vi "kf_update.vi"(8 "z":T1, 9 "u":T1, 11 "KF in":T2={"A"=[], "B"=[], "H"=[], "Q"=[], "R"=[], "x"=[], "P"=[], "x lim"=[], "y lim"=[], "K"=[], "Converge count"=-1} {"K" format="%#_3g"; "y lim" format="%#_3g"; "x lim" format="%#_3g"; "P" format="%#_3g"; "H" format="%#_3g"; "x" format="%#_3g"; "Q" format="%#_3g"; "R" format="%#_3g"; "B" format="%#_3g"; "A" format="%#_3g"}) -> (0 "y":T1, 3 "KF out":T2={"A"=[], "B"=[], "H"=[], "Q"=[], "R"=[], "x"=[], "P"=[], "x lim"=[], "y lim"=[], "K"=[], "Converge count"=-1} {"K" format="%#_3g"; "y lim" format="%#_3g"; "x lim" format="%#_3g"; "P" format="%#_3g"; "H" format="%#_3g"; "x" format="%#_3g"; "Q" format="%#_3g"; "R" format="%#_3g"; "B" format="%#_3g"; "A" format="%#_3g"})   [LabVIEW 2014]
uses:
  <vilib>/Analysis/Matrix/Datatypes/RealMatrix.ctl
  kalman_filter.ctl
  <vilib>/Analysis/baseanly.llb/Real A x B.vi
  <vilib>/Analysis/Matrix/Numeric/Add/Add - RM,RM.vi
  <vilib>/Analysis/Matrix/Numeric/Subtract/Subtract - RM,RM.vi
  <vilib>/Analysis/NI_AALBase.lvlib
  <vilib>/Analysis/Matrix/NI_Matrix.lvlib
panel:
  # "Command input.  If empty, this is the same as an appropriate dimension matrix of zeros."
  # "Measurement residue"
  # "Measurement."
  # "Something not exactly standard here is that the state (x) is a 2D array.  In the case where there is only one column, then this degenerates to the standard KF.  If there are multiple columns, then each column is an independent filter with identical structure and parameters (sometimes called block update).  When there are many independent axes this is significantly more efficient than the standard approach of concatenating independent systems on the diagonal.  It's also clearer because the parameter matrices end up much smaller, with fewer zero entries and less duplicated structure.\n\nBecause of this, the command input (u) and the measurement (z) are also 2D, with each column being the command or measurements for the corresponding filter."
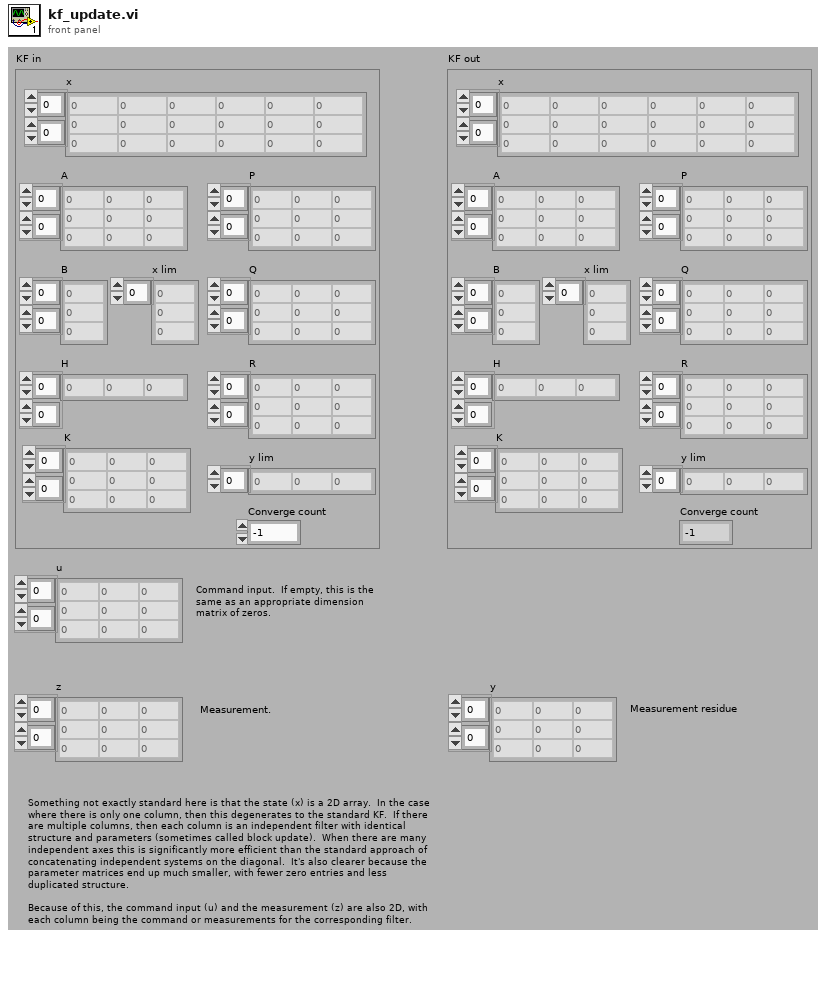
[diagram p1: front panel]
types:
  T1 = typedef "NI_Matrix.lvlib/RealMatrix.ctl" = dbl[][]
  T2 = typedef "kalman_filter.ctl" = cluster{"A":T1, "B":T1, "H":T1, "Q":T1, "R":T1, "x":T1, "P":T1, "x lim":dbl[], "y lim":dbl[], "K":T1, "Converge count":i32}
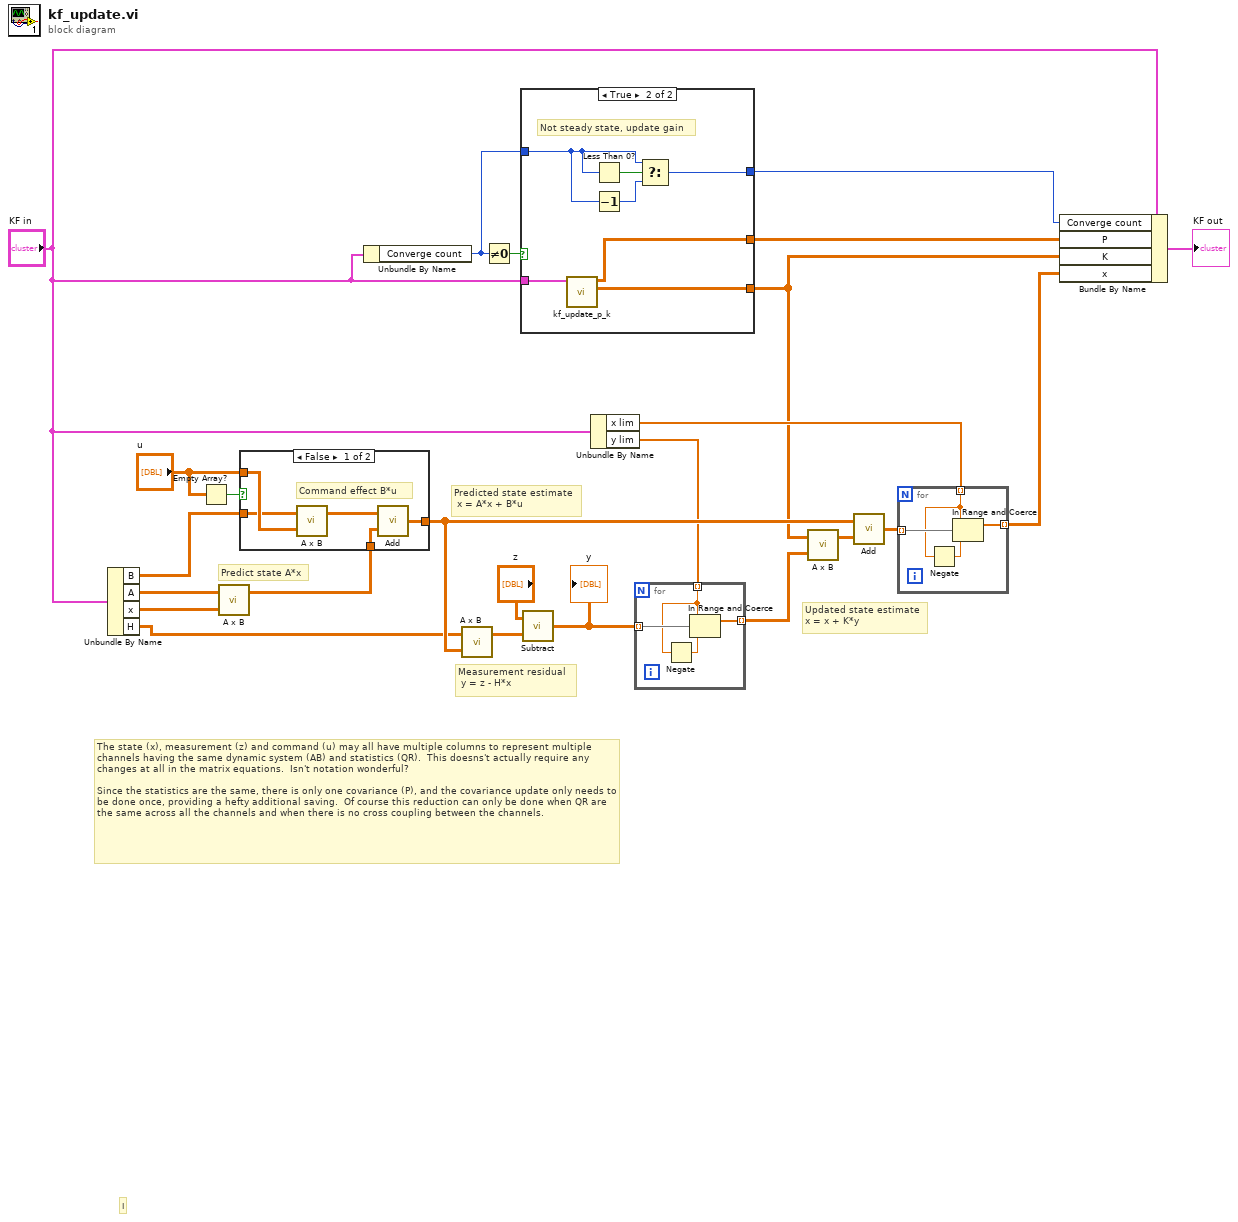
[diagram p0: block diagram]
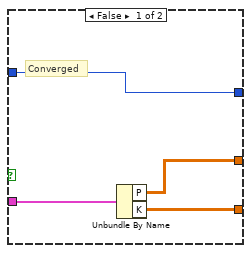
[diagram p2: hidden frame]
diagram:
  # "The state (x), measurement (z) and command (u) may all have multiple columns to represent multiple channels having the same dynamic system (AB) and statistics (QR).  This doesns't actually require any changes at all in the matrix equations.  Isn't notation wonderful?  \n\nSince the statistics are the same, there is only one covariance (P), and the covariance update only needs to be done once, providing a hefty additional saving.  Of course this reduction can only be done when QR are the same across all the channels and when there is no cross coupling between the channels."
  # "Updated state estimate\nx = x + K*y"
  # "Measurement residual\n y = z - H*x"
  # "Predicted state estimate\n x = A*x + B*u"
  # "Predict state A*x"
  # "I"
  n1 = Unbundle By Name("KF in") -> ("B"=w15:T1, "A"=w16:T1, "x"=w17:T1, "H"=w14:T1)
  n2 = Empty Array?(array="u") -> (empty?=w7:bool)
  n3 = call-poly <vilib>:"A x B.vi"("B"=w17, "A"=w16) -> ("A x B"=w20:T1)  [unwired: 1 out]
  n4 = case shown="False" w7 {
    tunnel: [w28 w30] -> w22
    tunnel: "u" -> [w27 _]
    tunnel: w20 -> [w26 w30]
    tunnel: w15 -> [w25 _]
    frame False {
      # "Command effect B*u"
      n5 = call-poly <vilib>:"A x B.vi"("B"=w27, "A"=w25) -> ("A x B"=w29:T1)  [unwired: 1 out]
      n6 = call-poly <vilib>:"Add.vi"("Real Matrix B"=w26, "Real Matrix A"=w29) -> ("A + B"=w28:T1)
    }
    frame True {
    }
  }
  n7 = Unbundle By Name("KF in") -> ("Converge count"=w3:i32)
  n8 = call-poly <vilib>:"A x B.vi"("B"=w22, "A"=w14) -> ("A x B"=w23:T1)  [unwired: 1 out]
  n9 = Not Equal To 0?(x=w3) -> (x != 0?=w4:bool)
  n10 = case shown="True" w4 {
    tunnel: [w33 w41] -> w1
    tunnel: [w32 w40] -> w19
    tunnel: "KF in" -> [w31 w39]
    tunnel: w3 -> [w34 w36]
    tunnel: [w34 w35] -> w2
    frame False {
      # "Converged"
      n11 = Unbundle By Name(w31) -> ("P"=w32:T1, "K"=w33:T1)
    }
    frame True {
      # "Not steady state, update gain"
      n12 = call "kf_update_p_k.vi"("KF in"=w39) -> ("K"=w41:T1, "P"=w40:T1)  [unwired: 9 in]
      n13 = Less Than 0?(x=w36) -> (x < 0?=w38:bool)
      n14 = Decrement(x=w36) -> (x-1=w37:i32)
      n15 = Select(t=w36, s=w38, f=w37) -> (s? t:f=w35:i32)
    }
  }
  n16 = call-poly <vilib>:"Subtract.vi"("Real Matrix B"=w23, "Real Matrix A"="z") -> ("A - B"=w11:T1)
  "y" <- w11
  n17 = Unbundle By Name("KF in") -> ("x lim"=w8:dbl[], "y lim"=w13:dbl[])
  n18 = for {
    tunnel: w11 -> [w45] mode=indexing
    tunnel: w13 -> [w44] mode=indexing
    tunnel: [w42] -> w12 mode=indexing
    n19 = Negate(x=w44) -> (-x=w43:dbl)
    n20 = In Range and Coerce(upper limit=w44, x=w45, lower limit=w43) -> (coerced(x)=w42:dbl[])  [unwired: 1 out]
  }
  n21 = call-poly <vilib>:"A x B.vi"("B"=w12, "A"=w1) -> ("A x B"=w21:T1)  [unwired: 1 out]
  n22 = call-poly <vilib>:"Add.vi"("Real Matrix B"=w21, "Real Matrix A"=w22) -> ("A + B"=w10:T1)
  n23 = for {
    tunnel: w10 -> [w49] mode=indexing
    tunnel: w8 -> [w48] mode=indexing
    tunnel: [w46] -> w9 mode=indexing
    n24 = Negate(x=w48) -> (-x=w47:dbl)
    n25 = In Range and Coerce(upper limit=w48, x=w49, lower limit=w47) -> (coerced(x)=w46:dbl[])  [unwired: 1 out]
  }
  n26 = Bundle By Name(cluster="KF in", "Converge count"=w2, "P"=w19, "K"=w1, "x"=w9) -> (→"KF out":T2)
